vi "TCP IP Parse CoagPower.vi"(11 "JSON in":string) -> (2 "Coag Power":string, 3 "JSON out":string)   [LabVIEW 2015]
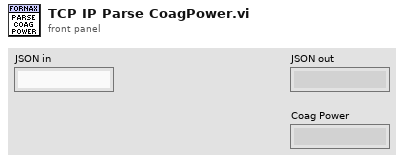
[diagram p1: front panel]
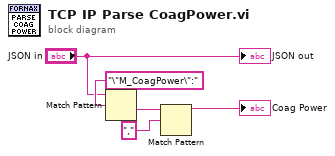
[diagram p0: block diagram]
diagram:
  n1 = Match Pattern(string="JSON in", regular expression="\"M_CoagPower\":") -> (after substring=w3:string)  [unwired: 1 in, 3 out]
  n2 = Match Pattern(string=w3, regular expression=",") -> (before substring=→"Coag Power":string)  [unwired: 1 in, 3 out]
  "JSON out" <- "JSON in"
